vi "Populate Bookmarks.vi"(8 "Error In":errorcluster, 10 "Scope":string="Main Application Instance", 11 "State In":T1) -> (0 "Error Out":errorcluster, 3 "State Out":T1)   [LabVIEW 2017, in "Graveyard.lvlib"]
uses:
  Graveyard.lvlib
  State.ctl
  Bookmarks Type.ctl
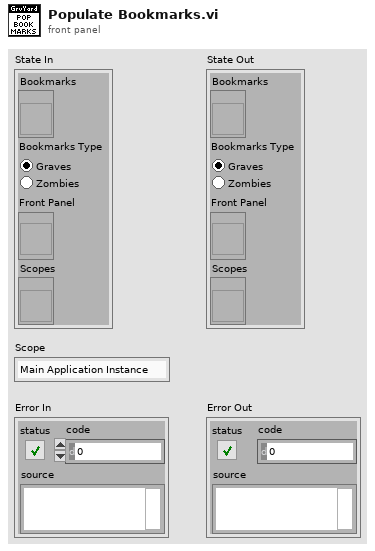
[diagram p1: front panel]
types:
  T1 = typedef "Graveyard.lvlib/State.ctl" = cluster{"Bookmarks":refnum<vi>, "Bookmarks Type":T2, "Front Panel":refnum<vi>, "Scopes":refnum<vi>}
  T2 = typedef "Graveyard.lvlib/Bookmarks Type.ctl" = enum32{"Graves", "Zombies"}
  T3 = enum8{"Enabled", "Disabled", "Disabled and Grayed Out"}
  T4 = typedef "Graveyard.lvlib/VI Information.ctl" = cluster{"App Info":T5, "Name":string, "Path":path}
  T5 = typedef "Graveyard.lvlib/Application Information.ctl" = cluster{"Project":string, "Target":string}
  T6 = typedef "Graveyard.lvlib/VI Bookmark.ctl" = cluster{"Bookmark Info":cluster{"Bookmark ID":u32, "Bookmark Tag":string, "Label Text":string}, "VI Info":T4}
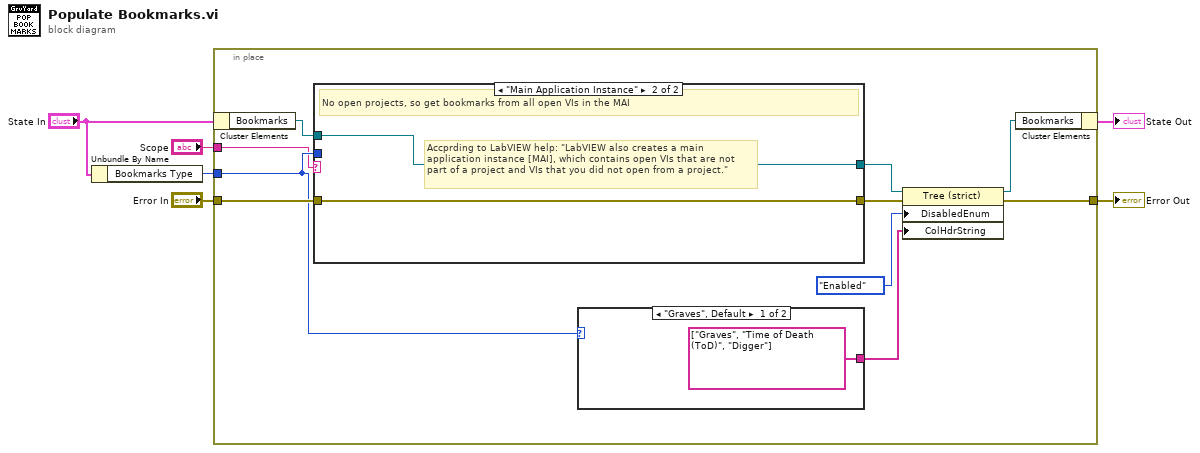
[diagram p0: block diagram]
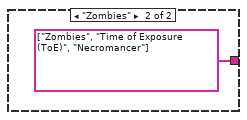
[diagram p2: hidden frame]
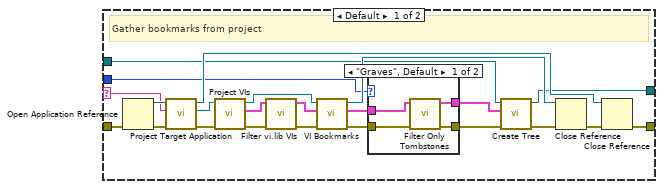
[diagram p3: hidden frame]
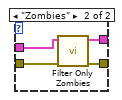
[diagram p4: hidden frame]
diagram:
  n1 = Unbundle By Name("State In") -> ("Bookmarks Type"=w2:T2)
  n2 = in-place {
    in-place-border: "Error In" -> [w16]
    in-place-border: [w13] -> w4
    in-place-border: w2 -> [w10]
    in-place-border: "Scope" -> [w8]
    n3 = in-place-cluster #1("State In") -> ("Bookmarks"=w14:refnum<vi>)
    n4 = case shown="\"Main Application Instance\"" w8 {
      selector: w8 -> [w38 _]
      tunnel: w16 -> [w41 w51]
      tunnel: [w37 w51] -> w15
      tunnel: w14 -> [w24 w50]
      tunnel: [w22 w50] -> w12
      tunnel: w10 -> [w19 _]
      frame Default {
        # "Gather bookmarks from project"
        n5 = Open Application Reference(8:w41) -> (0:w39:errorcluster, 3:w40:refnum<vi>)  [unwired: 3 in]
        n6 = call "Project Target Application.vi"("Error In"=w39, "Project Name"=w38, "App In"=w40) -> ("Error Out"=w35:errorcluster, "Project Target App"=w34:refnum<vi>, "App Out"=w36:refnum<vi>)  [unwired: 6 in]
        n7 = call "Project VIs.vi"("Error In"=w35, "Proejct Target App In"=w34) -> ("Error Out"=w31:errorcluster, "VIs"=w32:T4[], "Project Target App Out"=w28:refnum<vi>)  [unwired: 7 in]
        n8 = call "Filter vi.lib VIs.vi"("Error In"=w31, "VIs In"=w32) -> ("Error Out"=w30:errorcluster, "VIs Out"=w29:T4[])  [unwired: 8 in]
        n9 = call "VI Bookmarks.vi"("Error In"=w30, "VIs"=w29, "Project Target App In"=w28) -> ("Error Out"=w25:errorcluster, "VI Bookmarks"=w26:T6[], "Project Target App Out"=w27:refnum<vi>)  [unwired: 6 in]
        n10 = case shown="\"Graves\", Default" w19 {
          tunnel: w26 -> [w45 w49]
          tunnel: w25 -> [w44 w46]
          tunnel: [w43 w47] -> w23
          tunnel: [w42 w48] -> w20
          frame "Graves", Default {
            n11 = call "Filter Only Tombstones.vi"("Error In"=w44, "VI Bookmarks"=w45) -> ("Error Out"=w43:errorcluster, "Graves"=w42:T6[])  [unwired: 8 in]
          }
          frame "Zombies" {
            n12 = call "Filter Only Zombies.vi"("Error In"=w46, "VI Bookmarks"=w49) -> ("Error Out"=w47:errorcluster, "Zombies"=w48:T6[])  [unwired: 8 in]
          }
        }
        n13 = call "Create Tree.vi"("Error In"=w23, "Graves"=w20, "TreeControl In"=w24) -> ("Error Out"=w21:errorcluster, "TreeControl Out"=w22:refnum<vi>)  [unwired: 7 in]
        n14 = Close Reference(reference=w27, error in (no error)=w21) -> (error out=w33:errorcluster)
        n15 = Close Reference(reference=w36, error in (no error)=w33) -> (error out=w37:errorcluster)
      }
      frame "Main Application Instance" {
        # "Accprding to LabVIEW help: \"LabVIEW also creates a main application instance [MAI], which contains open VIs that are not part of a project and VIs that you did not open from a project.\""
        # "No open projects, so get bookmarks from all open VIs in the MAI"
      }
    }
    n16 = case shown="\"Graves\", Default" w10 {
      tunnel: [string[] ["Graves", "Time of Death (ToD)", "Digger"] string[] ["Zombies", "Time of Exposure (ToE)", "Necromancer"]] -> w9
      frame "Graves", Default {
      }
      frame "Zombies" {
      }
    }
    n17 = property class="Tree (strict)"(reference=w12, error in=w15, "DisabledEnum"=T3."Enabled" ("Disabled"), "ColHdrString"=w9) -> (reference out=w11:refnum<vi>, error out=w13:errorcluster)
    n18 = in-place-cluster #1("Bookmarks"=w11) -> (→"State Out":T1)
  }
  "Error Out" <- w4
